vi "室外Otsu.vi"(11 "火焰占比系数":dbl(slide)=0.9 min=0.0 max=1.0 step=0.01 scale=0.0..1.0 scale format="%1.2f") -> ()   [LabVIEW 2018]
doc: "This example shows how to open, read, and display an AVI file in NI Vision. The VI reads the frames per second property and plays the images back at the rate specified by the AVI file."
uses:
  <vilib>/vision/NI_Vision_Development_Module.lvlib
  Dll/fire_Otsu.dll
panel:
  in  "保存":bool
  out "像素当量单位":string
  out "像素当量":string
  in  "清除叠加火焰":bool
  out "总像素":dbl
  out "叠加像素源":u8[][](array[numeric])
  in  "暂停按钮":bool
  out "帧数据":T1
  out "导入像素当量":bool
  in  "火焰详细参数":bool
  out "叠加实际字符串":string
  out "单帧实际字符串":string
  out "叠加像素字符串":string
  out "单帧像素字符串":string
  out "火焰帧数":string
  out "叠加部分":string
  out "单帧部分":string
  in  "单帧回看":bool
  in  "返回":bool
  out "火焰分割":T2(plugin-control)
  out "单幅画面":T2(plugin-control) caption="单帧画面"
  in  "帧数计数":i32(slide) max=241 scale=-1.1..241.0
  in  "程序停止":bool
  out "原图":T2(plugin-control)
  out "火焰叠加":T2(plugin-control)
  # "基于Otsu的最大类间方法火焰分割"
  # "火焰参数"
  # "参\n数\n设\n置"
  # "说明：\n火焰实际面积的单位为标定时的设定的单位，若未进行标注，则不显示实际尺寸。"
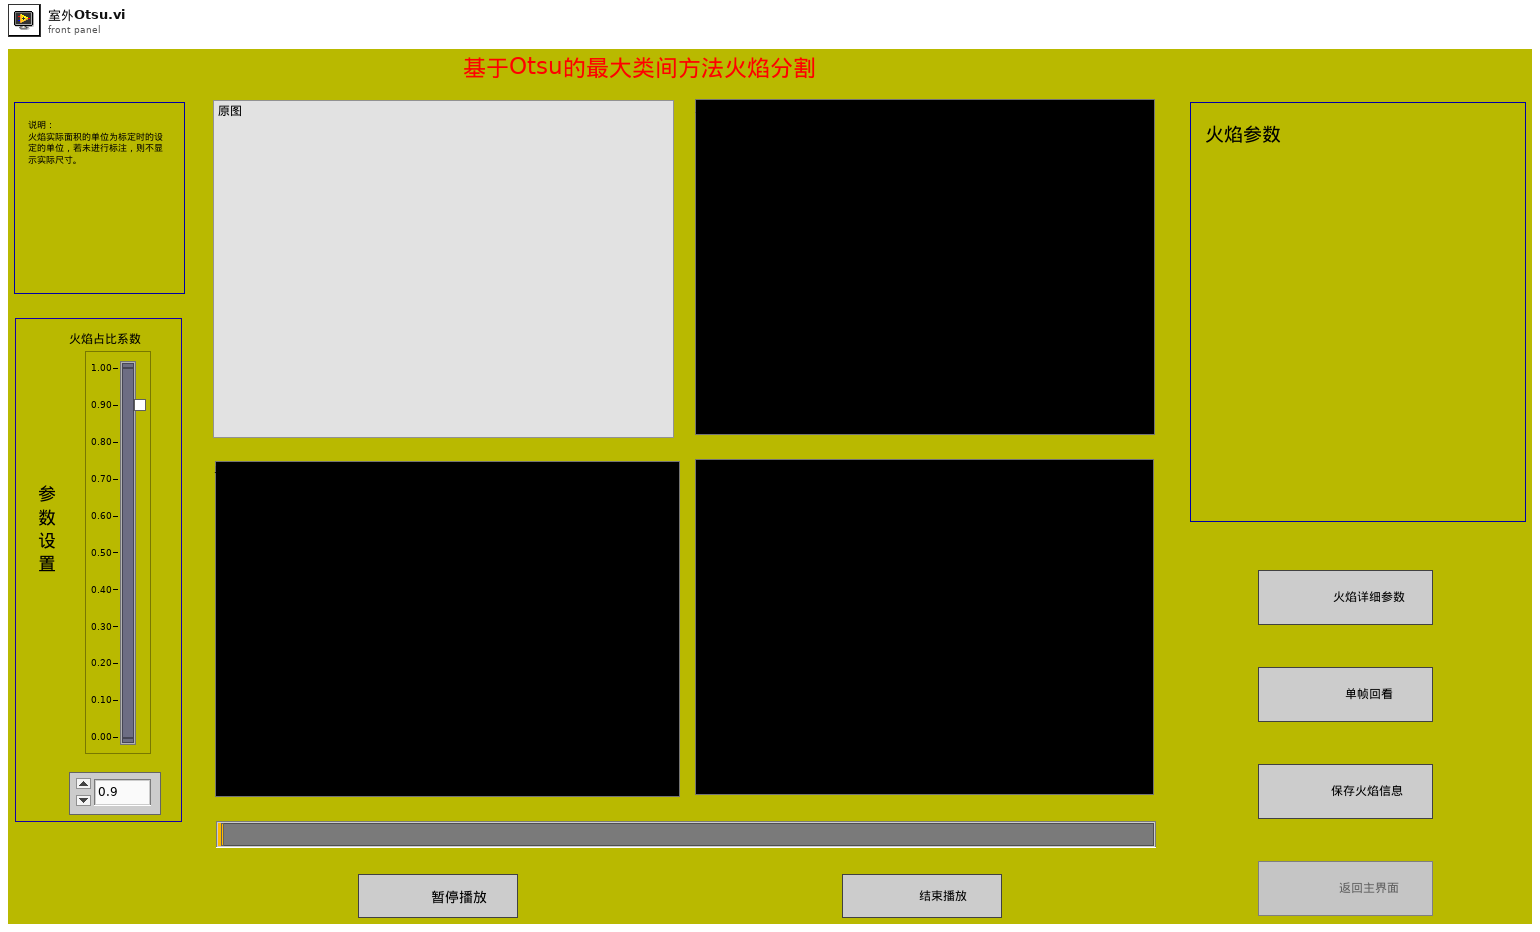
[diagram p1: front panel]
types:
  T1 = cluster{"Width":u32, "Height":u32, "Frames Per Second":u32, "Codec":string, "Has Data":bool}
  T2 = typedef "IMAQ Image.ctl" = refnum<image>
  T3 = enum8{"Enabled", "Disabled", "Disabled and Grayed Out"}
  T4 = typedef "Image Type" = u32
  T5 = enum32{"Invalid", "Standard", "Closed", "Hidden", "Minimized", "Maximized"}
  T6 = typedef "IMAQ AVI2 Refnum.ctl" = refnum<k20>
  T7 = cluster{"X Size":i32, "Y Size":i32, "% Tolerance":i32}
  T8 = typedef "ROI Descriptor" = cluster{"Global Rectangle":i32[], "Contours":cluster{"ID":enum32{"External", "Internal"}, "Type":u32, "Coordinates":i32[]}[]}
  T9 = cluster{"Area":dbl, "Number of Holes":dbl, "Bounding Rect":cluster{"Left":dbl, "Top":dbl, "Right":dbl, "Bottom":dbl}, "Center of Mass":cluster{"X":dbl, "Y":dbl}, "Orientation":dbl, "Dimensions":cluster{"Width":dbl, "Height":dbl}}[]
  T10 = cluster{"Particle Reports (Pixels)[0]":cluster{"Area":dbl, "Number of Holes":dbl, "Bounding Rect":cluster{"Left":dbl, "Top":dbl, "Right":dbl, "Bottom":dbl}, "Center of Mass":cluster{"X":dbl, "Y":dbl}, "Orientation":dbl, "Dimensions":cluster{"Width":dbl, "Height":dbl}}, "Particle Reports (Pixels)[1]":cluster{"Area":dbl, "Number of Holes":dbl, "Bounding Rect":cluster{"Left":dbl, "Top":dbl, "Right":dbl, "Bottom":dbl}, "Center of Mass":cluster{"X":dbl, "Y":dbl}, "Orientation":dbl, "Dimensions":cluster{"Width":dbl, "Height":dbl}}, "Particle Reports (Pixels)[2]":cluster{"Area":dbl, "Number of Holes":dbl, "Bounding Rect":cluster{"Left":dbl, "Top":dbl, "Right":dbl, "Bottom":dbl}, "Center of Mass":cluster{"X":dbl, "Y":dbl}, "Orientation":dbl, "Dimensions":cluster{"Width":dbl, "Height":dbl}}, "Particle Reports (Pixels)[3]":cluster{"Area":dbl, "Number of Holes":dbl, "Bounding Rect":cluster{"Left":dbl, "Top":dbl, "Right":dbl, "Bottom":dbl}, "Center of Mass":cluster{"X":dbl, "Y":dbl}, "Orientation":dbl, "Dimensions":cluster{"Width":dbl, "Height":dbl}}, "Particle Reports (Pixels)[4]":cluster{"Area":dbl, "Number of Holes":dbl, "Bounding Rect":cluster{"Left":dbl, "Top":dbl, "Right":dbl, "Bottom":dbl}, "Center of Mass":cluster{"X":dbl, "Y":dbl}, "Orientation":dbl, "Dimensions":cluster{"Width":dbl, "Height":dbl}}, "Particle Reports (Pixels)[5]":cluster{"Area":dbl, "Number of Holes":dbl, "Bounding Rect":cluster{"Left":dbl, "Top":dbl, "Right":dbl, "Bottom":dbl}, "Center of Mass":cluster{"X":dbl, "Y":dbl}, "Orientation":dbl, "Dimensions":cluster{"Width":dbl, "Height":dbl}}, "Particle Reports (Pixels)[6]":cluster{"Area":dbl, "Number of Holes":dbl, "Bounding Rect":cluster{"Left":dbl, "Top":dbl, "Right":dbl, "Bottom":dbl}, "Center of Mass":cluster{"X":dbl, "Y":dbl}, "Orientation":dbl, "Dimensions":cluster{"Width":dbl, "Height":dbl}}, "Particle Reports (Pixels)[7]":cluster{"Area":dbl, "Number of Holes":dbl, "Bounding Rect":cluster{"Left":dbl, "Top":dbl, "Right":dbl, "Bottom":dbl}, "Center of Mass":cluster{"X":dbl, "Y":dbl}, "Orientation":dbl, "Dimensions":cluster{"Width":dbl, "Height":dbl}}, "Particle Reports (Pixels)[8]":cluster{"Area":dbl, "Number of Holes":dbl, "Bounding Rect":cluster{"Left":dbl, "Top":dbl, "Right":dbl, "Bottom":dbl}, "Center of Mass":cluster{"X":dbl, "Y":dbl}, "Orientation":dbl, "Dimensions":cluster{"Width":dbl, "Height":dbl}}}
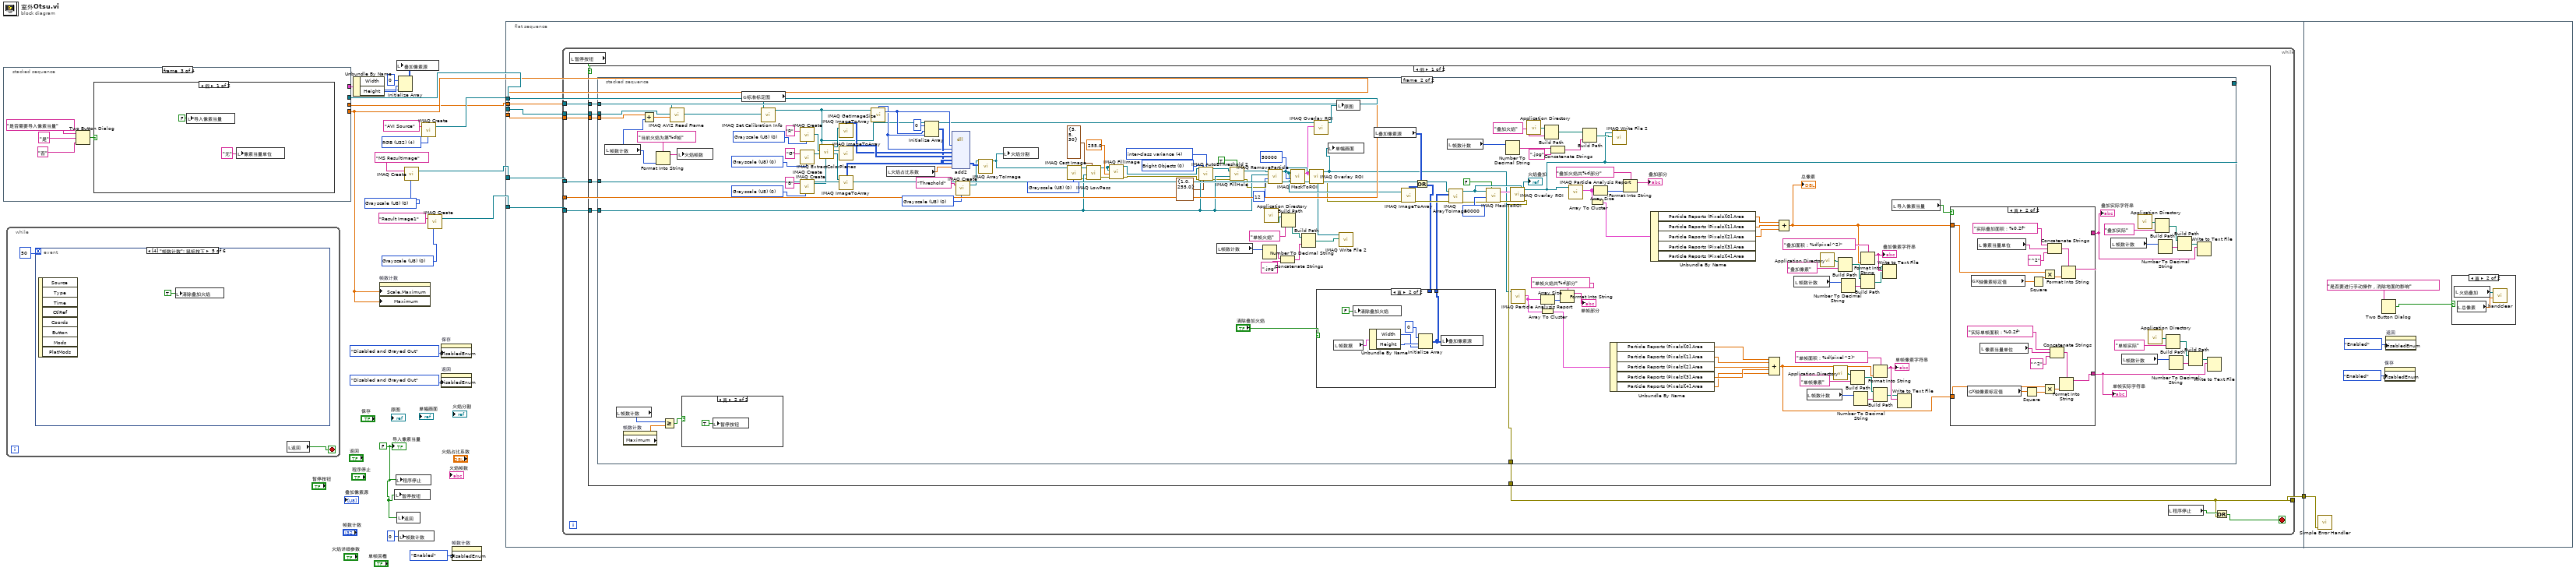
[diagram p0: block diagram]
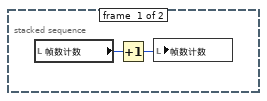
[diagram p2: hidden frame]
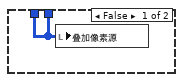
[diagram p3: hidden frame]
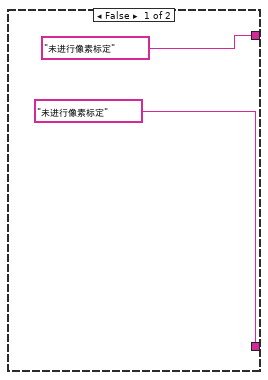
[diagram p5: hidden frame]
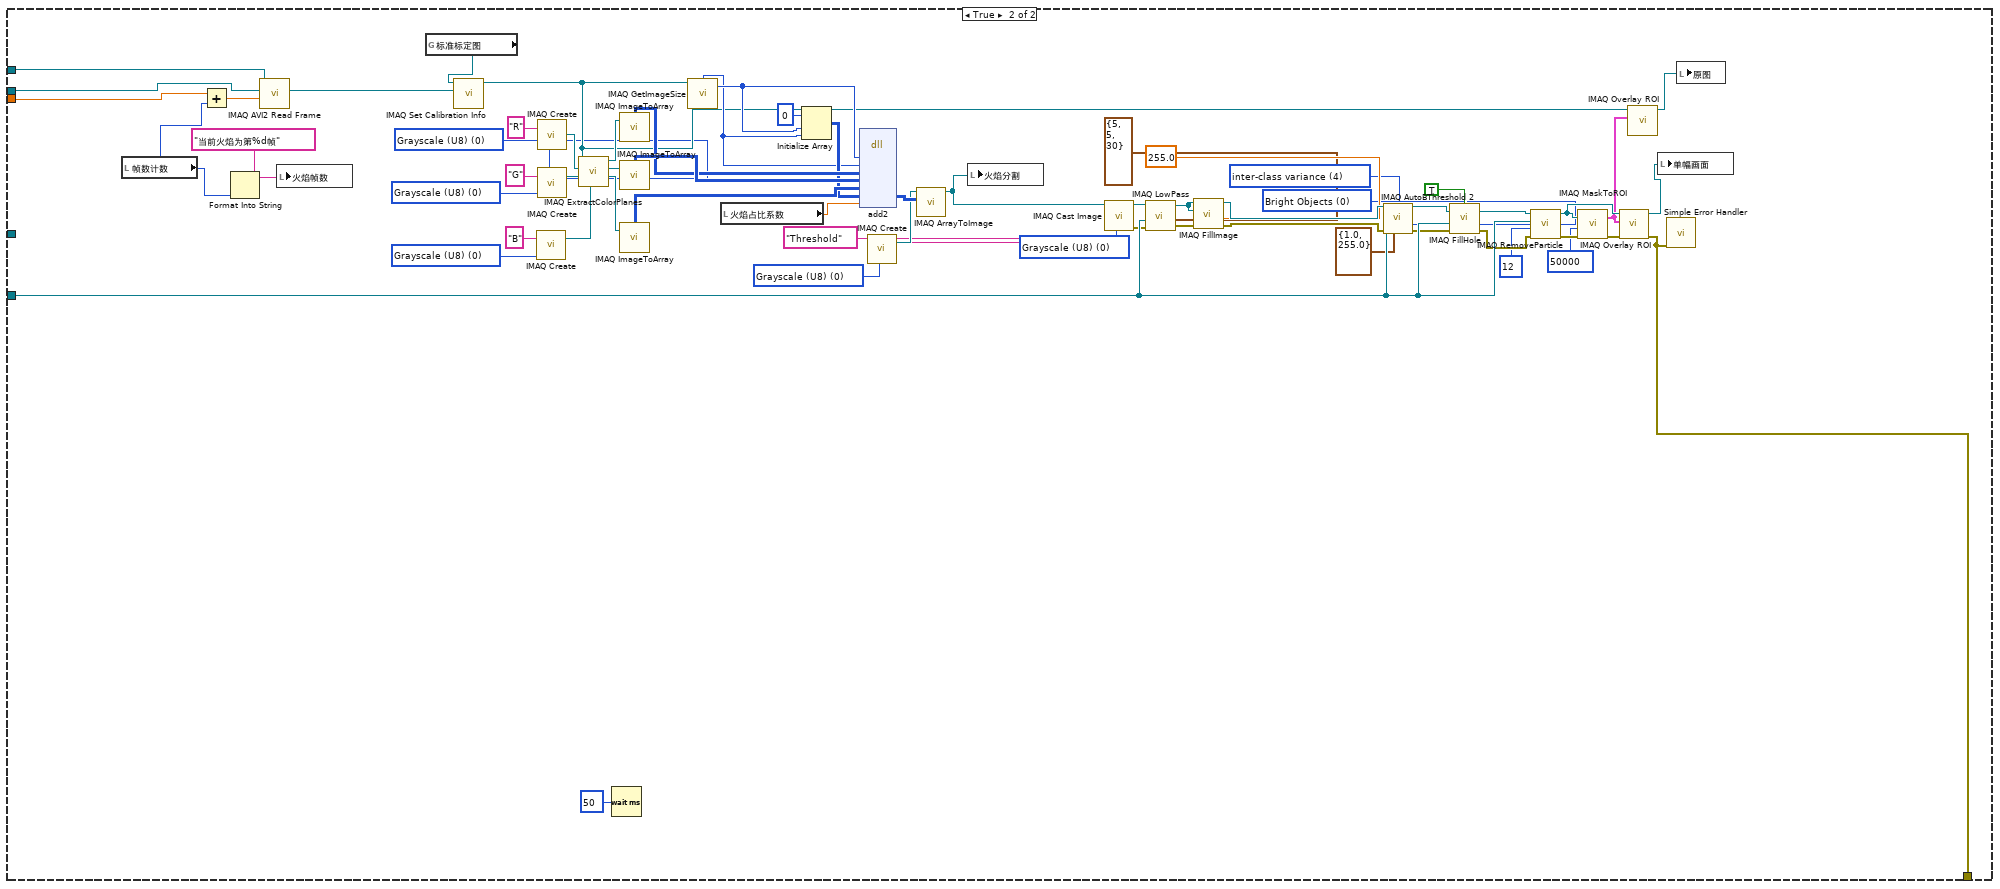
[diagram p6: hidden frame]
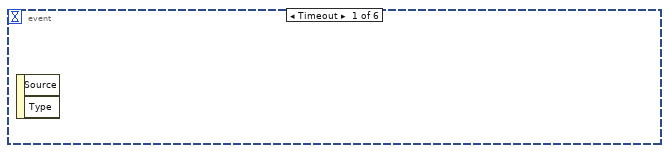
[diagram p8: hidden frame]
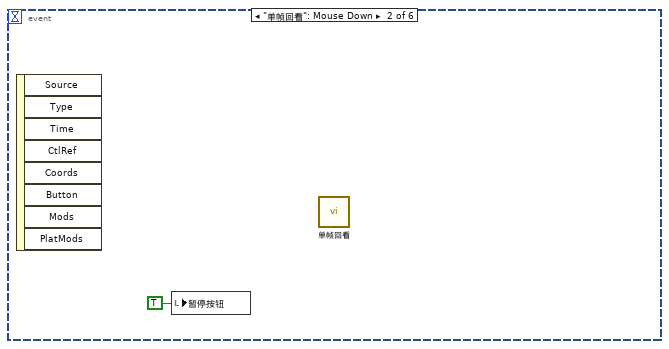
[diagram p9: hidden frame]
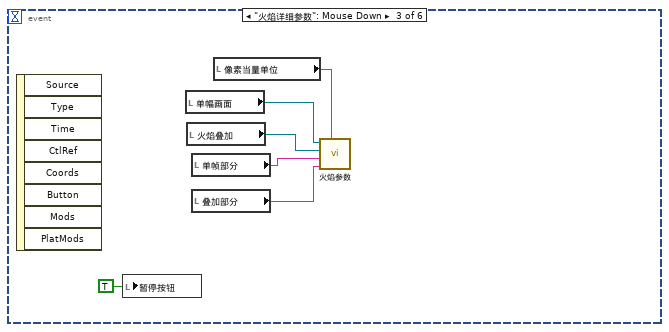
[diagram p10: hidden frame]
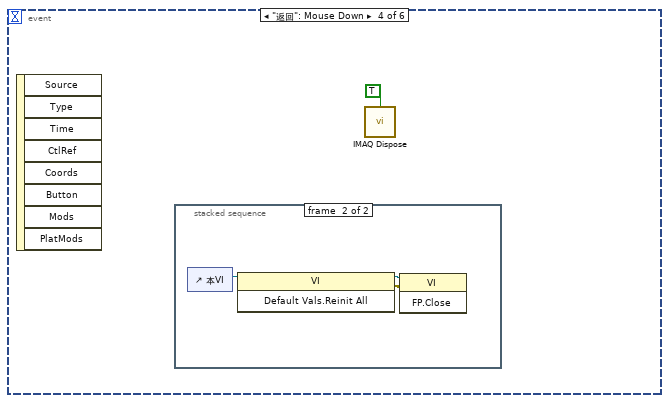
[diagram p11: hidden frame]
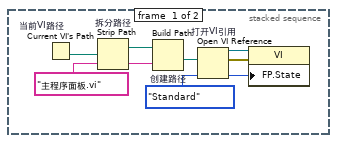
[diagram p12: hidden frame]
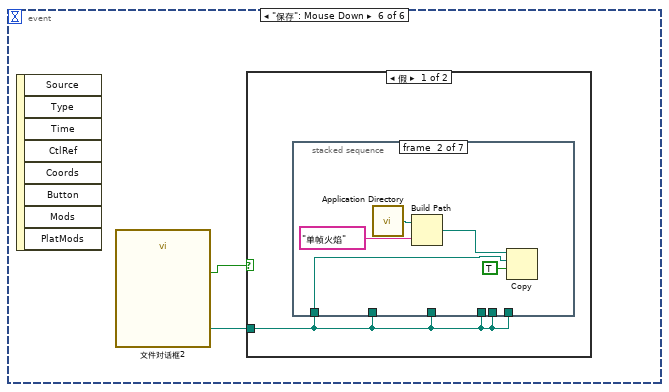
[diagram p13: hidden frame]
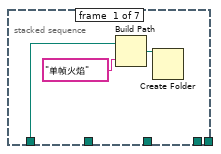
[diagram p14: hidden frame]
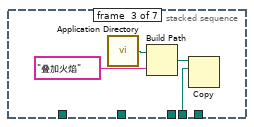
[diagram p15: hidden frame]
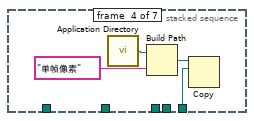
[diagram p16: hidden frame]
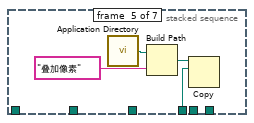
[diagram p17: hidden frame]
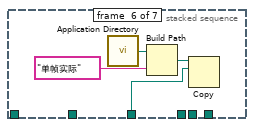
[diagram p18: hidden frame]
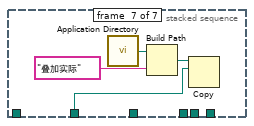
[diagram p19: hidden frame]
diagram:
  w17 = T4 0 items=["Grayscale (U8)", "Grayscale (I16)", "Grayscale (SGL)", "Complex (CSG)", "RGB (U32)", "HSL (U32)", "RGB (U64)", "Grayscale (U16)"] ("Image Type")
  w18 = T4 0 items=["Grayscale (U8)", "Grayscale (I16)", "Grayscale (SGL)", "Complex (CSG)", "RGB (U32)", "HSL (U32)", "RGB (U64)", "Grayscale (U16)"] ("Image Type")
  w20 = T4 4 items=["Grayscale (U8)", "Grayscale (I16)", "Grayscale (SGL)", "Complex (CSG)", "RGB (U32)", "HSL (U32)", "RGB (U64)", "Grayscale (U16)"] ("Image Type")
  w12 = FALSE ("导入像素当量")
  n1 = stacked-sequence {
    tunnel: [_ w31 _ _] -> w6
    tunnel: [_ w30 _ _] -> w5
    tunnel: [_ w29 _ _] -> w4
    tunnel: [_ w28 _ _] -> w22
    frame #0 {
      n2 = One Button Dialog(message="请选择室外火焰视频" ("消息"), button name ("OK")="确定" ("按钮名称（“确定”）")) -> ()  [unwired: 1 out]
    }
    frame #1 {
      n3 = control-ref of="本VI"() -> (w27:refnum<vi>)
      n4 = property class="VI"(reference=w27, "FP.State"=T5."Hidden" ("前面板窗口:状态")) -> ()  [unwired: 1 in, 2 out]
      n5 = call "帧数选择.vi"() -> ("AVI Refnum"=w31:T6, "初始帧"=w29:dbl, "Frame Data"=w28:T1, "结束帧"=w30:dbl)  [unwired: 5 in, 1 out]
      "帧数据" <- w28
    }
    frame #2 {
      n6 = Two Button Dialog(message="是否需要导入像素当量" ("消息"), 1:"否" ("F按钮名称（“取消”）"), 2:"是" ("T按钮名称（“确定”）")) -> (T button?=w32:bool)
      n7 = case shown="假" w32 {
        frame False {
          n8 = local write "导入像素当量"(FALSE ("导入像素当量")) -> ()
          n9 = local write "像素当量单位"("无" ("像素当量单位")) -> ()
        }
        frame True {
          n10 = stacked-sequence {
            frame #0 {
              n11 = call "文件对话框"("default name"="请选择像素当量") -> ("selected path"=w40:path)  [unwired: 11 in, 3 out]
              n12 = Read from Text File(file (use dialog)=w40) -> (text=w41:string)  [unwired: 3 in, 3 out]
              "像素当量" <- w41
              n13 = Fract/Exp String To Number(string=w41) -> (number=w42:dbl)  [unwired: 3 in, 1 out]
              n14 = local write "导入像素当量"(TRUE ("导入像素当量")) -> ()
              n15 = global write "全局变量.vi" "X轴像素标定值"(w42) -> ()
              n16 = global write "全局变量.vi" "Y轴像素标定值"(w42) -> ()
            }
            frame #1 {
              n17 = invoke on="像素当量" class="Str" method="Get Nth Line"("index"=u32 2 ("行索引")) -> (error out=w43:errorcluster, "text"=w44:string)  [unwired: 6 in, 5 out]
              n18 = case shown="错误" w43 {
                selector: w43 -> [_ w49]
                tunnel: w44 -> [w46 _]
                frame No Error {
                  "像素当量单位" <- w46
                }
                frame Error {
                  n19 = call <vilib>:"Simple Error Handler.vi"("error in (no error)"=w49) -> ()  [unwired: 4 in, 5 out]
                  n20 = local write "像素当量单位"("无" ("像素当量单位")) -> ()
                  n21 = One Button Dialog(message="导入像素当量单位时出错，\n请检查导入文件是否正确。" ("消息")) -> ()  [unwired: 1 in, 1 out]
                }
              }
            }
          }
        }
      }
    }
    frame #3 {
      n22 = flat-sequence {
        frame #0 {
          n23 = control-ref of="本VI"() -> (w51:refnum<vi>)
          n24 = property class="VI"(reference=w51, "FP.State"=T5."Standard" ("前面板窗口:状态")) -> ()  [unwired: 1 in, 2 out]
        }
        frame #1 {
          n25 = Wait (ms)(milliseconds to wait=u32 200 ("等待时间（毫秒）")) -> ()  [unwired: 1 out]
        }
      }
    }
  }
  n26 = while {
    stop <- w53 stop-if-true
    n27 = event "事件结构" shown="[4] \"帧数计数\": 鼠标按下" {
      selector: _ -> [_ _ _ _ _ _]
      dyn-events: _ -> [_ _ _ _ _ _]
      timeout: 50 -> [_ _ _ _ _ _]
      event Timeout {
        n28 = event-data() -> ()  [unwired: 1 in, 2 out]
      }
      event "单帧回看": Mouse Down {
        n29 = event-data() -> ()  [unwired: 1 in, 8 out]
        n30 = local write "暂停按钮"(TRUE ("暂停按钮")) -> ()
        n31 = call "单帧回看.vi"() -> ()  [unwired: 28 in]
      }
      event "火焰详细参数": Mouse Down {
        n32 = event-data() -> ()  [unwired: 1 in, 8 out]
        n33 = local write "暂停按钮"(TRUE ("暂停按钮")) -> ()
        n34 = local read "单幅画面"() -> (w59:T2)
        n35 = local read "火焰叠加"() -> (w58:T2)
        n36 = local read "单帧部分"() -> (w61:string)
        n37 = local read "叠加部分"() -> (w60:string)
        n38 = local read "像素当量单位"() -> (w56:string)
        n39 = call "火焰参数.vi"("像素当量单位"=w56, 8:w60, 9:w61, "Image 2"=w58, "Image"=w59) -> ()  [unwired: 7 in]
      }
      event "返回": Mouse Down {
        n40 = event-data() -> ()  [unwired: 1 in, 8 out]
        n41 = stacked-sequence {
          frame #0 {
            n42 = Current VI's Path "当前VI路径"() -> (path=w67:path)
            n43 = Strip Path "拆分路径"(path=w67) -> (stripped path=w69:path)  [unwired: 1 out]
            n44 = Build Path "创建路径"(base path=w69, name or relative path="主程序面板.vi" ("名称或相对路径")) -> (appended path=w68:path)
            n45 = Open VI Reference "打开VI引用"(vi path=w68) -> (vi reference=w66:refnum<vi>, error out=w65:errorcluster)  [unwired: 5 in]
            n46 = property class="VI"(reference=w66, error in=w65, "FP.State"=T5."Standard" ("前面板窗口:状态")) -> ()  [unwired: 2 out]
          }
          frame #1 {
            n47 = control-ref of="本VI"() -> (w70:refnum<vi>)
            n48 = invoke class="VI" method="Default Vals.Reinit All"(reference=w70) -> (reference out=w71:refnum<vi>, error out=w72:errorcluster)  [unwired: 2 in, 1 out]
            n49 = invoke class="VI" method="FP.Close"(reference=w71, error in=w72) -> ()  [unwired: 1 in, 3 out]
          }
        }
        n50 = call "IMAQ Dispose"("All Images? (No)"=TRUE) -> ()  [unwired: 2 in, 4 out]
      }
      event "帧数计数": Mouse Down {
        n51 = event-data() -> ()  [unwired: 1 in, 8 out]
        n52 = local write "清除叠加火焰"(TRUE ("清除叠加火焰")) -> ()
      }
      event "保存": Mouse Down {
        n53 = event-data() -> ()  [unwired: 1 in, 8 out]
        n54 = call "文件对话框2"() -> ("selected path"=w74:path, "cancelled"=w75:bool)  [unwired: 12 in, 2 out]
        n55 = case shown="假" w75 {
          tunnel: w74 -> [w76 _]
          frame False {
            n56 = stacked-sequence {
              tunnel: w76 -> [w77 w81 _ _ _ _ _]
              tunnel: w76 -> [_ _ w86 _ _ _ _]
              tunnel: w76 -> [_ _ _ w90 _ _ _]
              tunnel: w76 -> [_ _ _ _ w94 _ _]
              tunnel: w76 -> [_ _ _ _ _ w98 _]
              tunnel: w76 -> [_ _ _ _ _ _ w101]
              frame #0 {
                n57 = Build Path(base path=w77, name or relative path="单帧火焰" ("名称或相对路径")) -> (appended path=w79:path)
                n58 = Create Folder(path (use dialog)=w79) -> ()  [unwired: 2 in, 3 out]
              }
              frame #1 {
                n59 = call <vilib>:"Application Directory.vi"() -> ("Application Directory"=w84:path)
                n60 = Build Path(base path=w84, name or relative path="单帧火焰" ("名称或相对路径")) -> (appended path=w82:path)
                n61 = Copy(9:TRUE ("覆盖(F)"), 10:w81, 11:w82) -> ()  [unwired: 2 in, 3 out]
              }
              frame #2 {
                n62 = call <vilib>:"Application Directory.vi"() -> ("Application Directory"=w87:path)
                n63 = Build Path(base path=w87, name or relative path="叠加火焰" ("名称或相对路径")) -> (appended path=w88:path)
                n64 = Copy(10:w86, 11:w88) -> ()  [unwired: 3 in, 3 out]
              }
              frame #3 {
                n65 = call <vilib>:"Application Directory.vi"() -> ("Application Directory"=w91:path)
                n66 = Build Path(base path=w91, name or relative path="单帧像素" ("名称或相对路径")) -> (appended path=w92:path)
                n67 = Copy(10:w90, 11:w92) -> ()  [unwired: 3 in, 3 out]
              }
              frame #4 {
                n68 = call <vilib>:"Application Directory.vi"() -> ("Application Directory"=w95:path)
                n69 = Build Path(base path=w95, name or relative path="叠加像素" ("名称或相对路径")) -> (appended path=w96:path)
                n70 = Copy(10:w94, 11:w96) -> ()  [unwired: 3 in, 3 out]
              }
              frame #5 {
                n71 = call <vilib>:"Application Directory.vi"() -> ("Application Directory"=w99:path)
                n72 = Build Path(base path=w99, name or relative path="单帧实际" ("名称或相对路径")) -> (appended path=w100:path)
                n73 = Copy(10:w98, 11:w100) -> ()  [unwired: 3 in, 3 out]
              }
              frame #6 {
                n74 = call <vilib>:"Application Directory.vi"() -> ("Application Directory"=w103:path)
                n75 = Build Path(base path=w103, name or relative path="叠加实际" ("名称或相对路径")) -> (appended path=w104:path)
                n76 = Copy(10:w101, 11:w104) -> ()  [unwired: 3 in, 3 out]
              }
            }
          }
          frame True {
          }
        }
      }
    }
    n77 = local read "返回"() -> (w53:bool)
  }
  n78 = Unbundle By Name(w22) -> ("Width"=w14:u32, "Height"=w15:u32)
  n79 = property on="帧数计数" class="Slide (严格)"("Scale.Maximum"=w5, "Maximum"=w5) -> ()  [unwired: 2 in, 2 out]
  n80 = local write "暂停按钮"(w12) -> ()
  n81 = local write "程序停止"(w12) -> ()
  n82 = local write "返回"(w12) -> ()
  n83 = Initialize Array(u8 0 ("元素"), w15, w14) -> (w10:u8[][])
  n84 = local write "叠加像素源"(w10) -> ()
  n85 = local write "帧数计数"(0 ("帧数计数")) -> ()
  n86 = call "IMAQ Create"("Image Name"="MS ResultImage", "Image Type"=w17) -> ("New Image"=w7:T2)  [unwired: 2 in, 2 out]
  n87 = call "IMAQ Create"("Image Name"="AVI Source", "Image Type"=w20) -> ("New Image"=w9:T2)  [unwired: 2 in, 2 out]
  n88 = call "IMAQ Create"("Image Name"="Result Image1", "Image Type"=w18) -> ("New Image"=w8:T2)  [unwired: 2 in, 2 out]
  n89 = property on="保存" class="Bool (严格)"("DisabledEnum"=T3."Disabled and Grayed Out" ("禁用")) -> ()  [unwired: 2 in, 2 out]
  n90 = property on="返回" class="Bool (严格)"("DisabledEnum"=T3."Disabled and Grayed Out" ("禁用")) -> ()  [unwired: 2 in, 2 out]
  n91 = property on="帧数计数" class="Slide (严格)"("DisabledEnum"=T3."Enabled" ("禁用")) -> ()  [unwired: 2 in, 2 out]
  n92 = flat-sequence {
    tunnel: w9 -> [w111]
    tunnel: w8 -> [w110]
    tunnel: w7 -> [w109]
    tunnel: w6 -> [w108]
    tunnel: w5 -> [w107]
    tunnel: w4 -> [w106]
    tunnel: [w105] -> w3
    tunnel: w3 -> [w368]
    frame #0 {
      n93 = while {
        tunnel: w111 -> [w118]
        tunnel: w110 -> [w117]
        tunnel: w109 -> [w116]
        tunnel: w108 -> [w115]
        tunnel: w107 -> [_]
        tunnel: w106 -> [w120]
        tunnel: [w112] -> w105
        stop <- w113 stop-if-true
        n94 = local read "暂停按钮"() -> (w119:bool)
        n95 = case shown="假" w119 {
          tunnel: w116 -> [w126 _]
          tunnel: w117 -> [w125 w362]
          tunnel: w118 -> [w124 w364]
          tunnel: w115 -> [w123 w365]
          tunnel: w120 -> [w122 w363]
          tunnel: [w121 w304] -> w112
          frame False {
            n96 = stacked-sequence {
              tunnel: w126 -> [_ w275]
              tunnel: w125 -> [_ w274]
              tunnel: w124 -> [_ w273]
              tunnel: w123 -> [_ w149]
              tunnel: w122 -> [_ w148]
              tunnel: [_ w141] -> w121
              tunnel: [_ w137] -> _
              frame #0 {
                n97 = local read "帧数计数"() -> (w128:i32)
                n98 = Increment(x=w128) -> (x+1=w127:i32)
                n99 = local write "帧数计数"(w127) -> ()
              }
              frame #1 {
                w224 = T4 0 items=["Grayscale (U8)", "Grayscale (I16)", "Grayscale (SGL)", "Complex (CSG)", "RGB (U32)", "HSL (U32)", "RGB (U64)", "Grayscale (U16)"] ("Image Type")
                w231 = T4 0 items=["Grayscale (U8)", "Grayscale (I16)", "Grayscale (SGL)", "Complex (CSG)", "RGB (U32)", "HSL (U32)", "RGB (U64)", "Grayscale (U16)"] ("Image Type")
                w232 = T4 0 items=["Grayscale (U8)", "Grayscale (I16)", "Grayscale (SGL)", "Complex (CSG)", "RGB (U32)", "HSL (U32)", "RGB (U64)", "Grayscale (U16)"] ("Image Type")
                w233 = T4 0 items=["Grayscale (U8)", "Grayscale (I16)", "Grayscale (SGL)", "Complex (CSG)", "RGB (U32)", "HSL (U32)", "RGB (U64)", "Grayscale (U16)"] ("Image Type")
                w265 = u32 0 items=["Bright Objects", "Dark Objects"] ("Look For (Bright Objects)")
                w268 = 4 items=["clustering", "entropy", "metric", "moments", "inter-class variance"] ("Method")
                w269 = T4 0 items=["Grayscale (U8)", "Grayscale (I16)", "Grayscale (SGL)", "Complex (CSG)", "RGB (U32)", "HSL (U32)", "RGB (U64)", "Grayscale (U16)"] ("Image Type")
                n100 = local read "帧数计数"() -> (w147:i32)
                n101 = local read "帧数计数"() -> (w145:i32)
                n102 = property on="帧数计数" class="Slide (严格)"() -> ("Maximum"=w144:dbl)  [unwired: 2 in, 2 out]
                n103 = Add(x=w148, y=w147) -> (x+y=w219:dbl)
                n104 = Format Into String(format string="当前火焰为第%d帧" ("初始字符串"), w147) -> (resulting string=w136:string)  [unwired: 2 in, 1 out]
                n105 = Greater Or Equal?(x=w145, y=w144) -> (x >= y?=w143:bool)
                n106 = call "IMAQ AVI2 Read Frame"("Frame Number"=w219, "Image"=w273, "AVI Refnum"=w149) -> ("Image Out"=w197:T2)  [unwired: 1 in, 7 out]
                n107 = local write "火焰帧数"(w136) -> ()
                n108 = case shown="真" w143 {
                  frame False {
                  }
                  frame True {
                    n109 = local write "暂停按钮"(TRUE ("暂停按钮")) -> ()
                  }
                }
                n110 = global read "全局变量.vi" "标准标定图"() -> (w196:T2)
                n111 = call "IMAQ Set Calibration Info"("Image Dst"=w197, "Image Src"=w196) -> ("Calibrated Image"=w198:T2)  [unwired: 8 in, 1 out]
                n112 = call "IMAQ Create"("Image Name"="B", "Image Type"=w231) -> ("New Image"=w242:T2)  [unwired: 3 in, 1 out]
                n113 = call "IMAQ Create"("Image Name"="R", "Image Type"=w233) -> ("New Image"=w240:T2)  [unwired: 3 in, 1 out]
                n114 = call "IMAQ Create"("Image Name"="G", "Image Type"=w232) -> ("New Image"=w238:T2)  [unwired: 3 in, 1 out]
                n115 = call "IMAQ ExtractColorPlanes"("Blue or Luma or Val or Inten Plane"=w242, "Green or Sat Plane"=w238, "Red or Hue Plane"=w240, "Image Src"=w198) -> ("Blue or Luma or Val or Inten Plane out"=w234:T2, "Green or Sat Plane out"=w235:T2, "Red or Hue Plane out"=w236:T2)  [unwired: 4 in, 1 out]
                n116 = call "IMAQ ImageToArray"("Image"=w236) -> ("Image Pixels (U8)"=w228:u8[][])  [unwired: 3 in, 4 out]
                n117 = call "IMAQ ImageToArray"("Image"=w235) -> ("Image Pixels (U8)"=w230:u8[][])  [unwired: 3 in, 4 out]
                n118 = call "IMAQ ImageToArray"("Image"=w234) -> ("Image Pixels (U8)"=w229:u8[][])  [unwired: 3 in, 4 out]
                n119 = call "IMAQ GetImageSize"("Image"=w198) -> ("Y Resolution"=w221:i32, "X Resolution"=w220:i32)  [unwired: 3 in, 1 out]
                n120 = local read "火焰占比系数"() -> (w135:dbl)
                n121 = Initialize Array ("data")(u8 0, w221, w220) -> (w223:u8[][])
                n122 = dll-call lib="PTH2Aabs DsdhProgramme_GuShiJu火焰分割Dll\nfire_Otsu.dll" fn="add2"("rows"=w221, "cols"=w220, "ImageR"=w228, "ImageG"=w230, "ImageB"=w229, "data"=w223, "a"=w135) -> ("data"=w227:u8[][])  [unwired: 10 in, 2 out]
                n123 = call "IMAQ Create"("Image Name"="Threshold", "Image Type"=w224) -> ("New Image"=w226:T2)  [unwired: 3 in, 1 out]
                n124 = call "IMAQ ArrayToImage"("Image Pixels (U8)"=w227, "Image"=w226) -> ("Image Out"=w134:T2)  [unwired: 8 in, 1 out]
                n125 = local write "火焰分割"(w134) -> ()
                n126 = call "IMAQ Cast Image"("Image Type"=w269, "Image Src"=w134) -> ("error out"=w248:errorcluster, "Image Dst Out"=w244:T2)  [unwired: 8 in]
                n127 = call "IMAQ LowPass"("Image Src"=w244, "Size & Tolerance"=T7 {"X Size"=5, "Y Size"=5, "% Tolerance"=30}, "Image Dst"=w274, "error in (no error)"=w248) -> ("Image Dst Out"=w252:T2, "error out"=w256:errorcluster)  [unwired: 3 in]
                n128 = call "IMAQ FillImage"("error in (no error)"=w256, "Pixel Value (U8, U16, I16, Float)"=sgl 255.0, "Image Mask"=w252, "Image"=w252) -> ("error out"=w255:errorcluster, "Image Out"=w251:T2)  [unwired: 6 in]
                n129 = call "IMAQ AutoBThreshold 2"("Image Src"=w251, "Look For (Bright Objects)"=w265, "Method (clustering)"=w268, "Image Dst"=w274, "error in (no error)"=w255, "Threshold Limits"=cluster{"Lower value":sgl, "Upper value":sgl} {"Lower value"=1.0, "Upper value"=255.0}) -> ("Image Dst Out"=w254:T2, "error out"=w267:errorcluster)  [unwired: 2 in, 6 out]
                n130 = local read "帧数计数"() -> (w187:i32)
                n131 = call "IMAQ FillHole"("error in (no error)"=w267, "Image Dst"=w274, "Image Src"=w254, "Connectivity 4/8 (8)"=TRUE) -> ("error out"=w263:errorcluster, "Image Dst Out"=w253:T2)  [unwired: 2 in]
                n132 = Number To Decimal String(number=w187) -> (decimal integer string=w182:string)  [unwired: 1 in]
                n133 = call <vilib>:"Application Directory.vi"() -> ("Application Directory"=w195:path)
                n134 = call "IMAQ RemoveParticle"("error in (no error)"=w263, "Number of Erosion"=12, "Image Dst"=w274, "Image Src"=w253) -> ("error out"=w261:errorcluster, "Image Dst Out"=w250:T2)  [unwired: 6 in]
                n135 = Concatenate Strings(w182, ".jpg" ("字符串")) -> (w181:string)
                n136 = Build Path(base path=w195, name or relative path="单帧火焰" ("名称或相对路径")) -> (appended path=w194:path)
                n137 = call "IMAQ MaskToROI"("Image"=w250, "Max number of vectors in ROI"=50000, "error in (no error)"=w261) -> ("ROI Descriptor"=w200:T8, "error out"=w260:errorcluster)  [unwired: 4 in, 1 out]
                n138 = Build Path(base path=w194, name or relative path=w181) -> (appended path=w193:path)
                n139 = call "IMAQ Overlay ROI"("error in (no error)"=w260, "ROI Descriptor"=w200, "Image"=w250) -> ("error out"=w146:errorcluster, "Image Out"=w132:T2)  [unwired: 7 in]
                n140 = call "IMAQ Overlay ROI"("ROI Descriptor"=w200, "Image"=w198) -> ("Image Out"=w133:T2)  [unwired: 8 in, 1 out]
                n141 = local write "单幅画面"(w132) -> ()
                n142 = local write "原图"(w133) -> ()
                n143 = call-poly "IMAQ Write File 2"("File Path"=w193, "Image"=w132) -> ()  [unwired: 8 in, 2 out]
                n144 = local read "叠加像素源"() -> (w142:u8[][])
                n145 = call "IMAQ ImageToArray"("error in (no error)"=w146, "Image"=w250) -> ("error out"=w247:errorcluster, "Image Pixels (U8)"=w249:u8[][])  [unwired: 2 in, 3 out]
                n146 = Or(x=w142, y=w249) -> (x .or. y?=w131:u8[][])
                n147 = case shown="真" "清除叠加火焰" {
                  tunnel: w131 -> [w276 _]
                  tunnel: [w276 w278] -> w129
                  frame False {
                    n148 = local write "叠加像素源"(w276) -> ()
                  }
                  frame True {
                    n149 = local read "帧数据"() -> (w280:T1)
                    n150 = local write "清除叠加火焰"(FALSE ("清除叠加火焰")) -> ()
                    n151 = Unbundle By Name(w280) -> ("Width"=w281:u32, "Height"=w282:u32)
                    n152 = Initialize Array(0, w282, w281) -> (w278:i32[][])
                    n153 = local write "叠加像素源"(w278) -> ()
                  }
                }
                n154 = local read "帧数计数"() -> (w186:i32)
                n155 = call "IMAQ ArrayToImage"("error in (no error)"=w247, "Image Pixels (U8)"=w129, "Image"=w275) -> ("error out"=w246:errorcluster, "Image Out"=w245:T2)  [unwired: 7 in]
                n156 = call "IMAQ MaskToROI"("External edges only (T)"=FALSE, "Image"=w245, "Max number of vectors in ROI"=50000, "error in (no error)"=w246) -> ("ROI Descriptor"=w272:T8, "error out"=w271:errorcluster)  [unwired: 3 in, 1 out]
                n157 = Number To Decimal String(number=w186) -> (decimal integer string=w185:string)  [unwired: 1 in]
                n158 = call "IMAQ Overlay ROI"("error in (no error)"=w271, "ROI Descriptor"=w272, "Image"=w245) -> ("error out"=w141:errorcluster, "Image Out"=w137:T2)  [unwired: 7 in]
                "火焰叠加" <- w137
                n159 = call "IMAQ Particle Analysis Report"("Image"=w132) -> ("Particle Reports (Pixels)"=w205:T9)  [unwired: 5 in, 5 out]
                n160 = call <vilib>:"Application Directory.vi"() -> ("Application Directory"=w191:path)
                n161 = Array To Cluster(array=w205) -> (cluster=w218:T10)
                n162 = Array Size(array=w205) -> (size(s)=w208:i32)
                n163 = Build Path(base path=w191, name or relative path="叠加火焰" ("名称或相对路径")) -> (appended path=w189:path)
                n164 = Concatenate Strings(w185, ".jpg" ("字符串")) -> (w184:string)
                n165 = Format Into String(format string="单帧火焰共%d部分" ("初始字符串"), w208) -> (resulting string=→"单帧部分":string)  [unwired: 2 in, 1 out]
                n166 = call "IMAQ Particle Analysis Report"("Image"=w137) -> ("Particle Reports (Pixels)"=w201:T9)  [unwired: 5 in, 5 out]
                n167 = Build Path(base path=w189, name or relative path=w184) -> (appended path=w188:path)
                n168 = Array To Cluster(array=w201) -> (cluster=w214:T10)
                n169 = Array Size(array=w201) -> (size(s)=w203:i32)
                n170 = Unbundle By Name(w218) -> ("Particle Reports (Pixels)[0].Area"=w217:dbl, "Particle Reports (Pixels)[1].Area"=w216:dbl, "Particle Reports (Pixels)[2].Area"=w215:dbl, "Particle Reports (Pixels)[3].Area"=w213:dbl, "Particle Reports (Pixels)[4].Area"=w212:dbl)
                n171 = call-poly "IMAQ Write File 2"("File Path"=w188, "Image"=w137) -> ()  [unwired: 8 in, 2 out]
                n172 = Format Into String(format string="叠加火焰共%d部分" ("初始字符串"), w203) -> (resulting string=→"叠加部分":string)  [unwired: 2 in, 1 out]
                n173 = Unbundle By Name(w214) -> ("Particle Reports (Pixels)[0].Area"=w211:dbl, "Particle Reports (Pixels)[1].Area"=w210:dbl, "Particle Reports (Pixels)[2].Area"=w209:dbl)  [unwired: 2 out]
                n174 = Compound Arithmetic op=ADD(w217, w216, w215, w213, w212) -> (w140:dbl)
                n175 = Compound Arithmetic op=ADD(w211, w210, w209) -> (w138:dbl)
                "总像素" <- w138
                n176 = local read "帧数计数"() -> (w170:i32)
                n177 = local read "帧数计数"() -> (w174:i32)
                n178 = call <vilib>:"Application Directory.vi"() -> ("Application Directory"=w171:path)
                n179 = call <vilib>:"Application Directory.vi"() -> ("Application Directory"=w173:path)
                n180 = Build Path(base path=w171, name or relative path="叠加像素" ("字符串")) -> (appended path=w164:path)
                n181 = Number To Decimal String(number=w170) -> (decimal integer string=w162:string)  [unwired: 1 in]
                n182 = Build Path(base path=w173, name or relative path="单帧像素" ("字符串")) -> (appended path=w151:path)
                n183 = Number To Decimal String(number=w174) -> (decimal integer string=w150:string)  [unwired: 1 in]
                n184 = Format Into String(format string="叠加面积：%d(pixel^2)" ("格式字符串"), w138) -> (resulting string=w169:string)  [unwired: 2 in, 1 out]
                "叠加像素字符串" <- w169
                n185 = Build Path(base path=w164, name or relative path=w162) -> (appended path=w163:path)
                n186 = Format Into String(format string="单帧面积：%d(pixel^2)" ("格式字符串"), w140) -> (resulting string=w172:string)  [unwired: 2 in, 1 out]
                "单帧像素字符串" <- w172
                n187 = Build Path(base path=w151, name or relative path=w150) -> (appended path=w152:path)
                n188 = Write to Text File(file (use dialog)=w163, text=w169) -> ()  [unwired: 2 in, 3 out]
                n189 = local read "导入像素当量"() -> (w177:bool)
                n190 = Write to Text File(file (use dialog)=w152, text=w172) -> ()  [unwired: 2 in, 3 out]
                n191 = case shown="真" w177 {
                  tunnel: ["未进行像素标定" w303] -> w166
                  tunnel: w138 -> [_ w300]
                  tunnel: w140 -> [_ w295]
                  tunnel: ["未进行像素标定" w294] -> w139
                  frame False {
                  }
                  frame True {
                    n192 = global read "全局变量.vi" "X轴像素标定值"() -> (w297:dbl)
                    n193 = global read "全局变量.vi" "X轴像素标定值"() -> (w301:dbl)
                    n194 = local read "像素当量单位"() -> (w292:string)
                    n195 = local read "像素当量单位"() -> (w289:string)
                    n196 = Square(x=w297) -> (x^2=w296:dbl)
                    n197 = Square(x=w301) -> (x^2=w302:dbl)
                    n198 = Multiply(x=w300, y=w302) -> (x*y=w299:dbl)
                    n199 = Multiply(x=w295, y=w296) -> (x*y=w298:dbl)
                    n200 = Concatenate Strings("实际叠加面积：%0.2f" ("格式字符串"), w292, "^2" ("字符串")) -> (w290:string)
                    n201 = Concatenate Strings("实际单帧面积：%0.2f" ("格式字符串"), w289, "^2" ("字符串")) -> (w286:string)
                    n202 = Format Into String(format string=w286, w298) -> (resulting string=w294:string)  [unwired: 2 in, 1 out]
                    n203 = Format Into String(format string=w290, w299) -> (resulting string=w303:string)  [unwired: 2 in, 1 out]
                  }
                }
                "单帧实际字符串" <- w139
                "叠加实际字符串" <- w166
                n204 = local read "帧数计数"() -> (w168:i32)
                n205 = local read "帧数计数"() -> (w175:i32)
                n206 = call <vilib>:"Application Directory.vi"() -> ("Application Directory"=w167:path)
                n207 = call <vilib>:"Application Directory.vi"() -> ("Application Directory"=w176:path)
                n208 = Build Path(base path=w167, name or relative path="叠加实际" ("字符串")) -> (appended path=w161:path)
                n209 = Number To Decimal String(number=w168) -> (decimal integer string=w159:string)  [unwired: 1 in]
                n210 = Build Path(base path=w176, name or relative path="单帧实际" ("字符串")) -> (appended path=w157:path)
                n211 = Number To Decimal String(number=w175) -> (decimal integer string=w156:string)  [unwired: 1 in]
                n212 = Build Path(base path=w161, name or relative path=w159) -> (appended path=w158:path)
                n213 = Build Path(base path=w157, name or relative path=w156) -> (appended path=w154:path)
                n214 = Write to Text File(file (use dialog)=w158, text=w166) -> ()  [unwired: 2 in, 3 out]
                n215 = Write to Text File(file (use dialog)=w154, text=w139) -> ()  [unwired: 2 in, 3 out]
              }
            }
          }
          frame True {
            w320 = T4 0 items=["Grayscale (U8)", "Grayscale (I16)", "Grayscale (SGL)", "Complex (CSG)", "RGB (U32)", "HSL (U32)", "RGB (U64)", "Grayscale (U16)"] ("Image Type")
            w318 = T4 0 items=["Grayscale (U8)", "Grayscale (I16)", "Grayscale (SGL)", "Complex (CSG)", "RGB (U32)", "HSL (U32)", "RGB (U64)", "Grayscale (U16)"] ("Image Type")
            w314 = T4 0 items=["Grayscale (U8)", "Grayscale (I16)", "Grayscale (SGL)", "Complex (CSG)", "RGB (U32)", "HSL (U32)", "RGB (U64)", "Grayscale (U16)"] ("Image Type")
            w316 = T4 0 items=["Grayscale (U8)", "Grayscale (I16)", "Grayscale (SGL)", "Complex (CSG)", "RGB (U32)", "HSL (U32)", "RGB (U64)", "Grayscale (U16)"] ("Image Type")
            w308 = u32 0 items=["Bright Objects", "Dark Objects"] ("Look For (Bright Objects)")
            w307 = 4 items=["clustering", "entropy", "metric", "moments", "inter-class variance"] ("Method")
            w305 = T4 0 items=["Grayscale (U8)", "Grayscale (I16)", "Grayscale (SGL)", "Complex (CSG)", "RGB (U32)", "HSL (U32)", "RGB (U64)", "Grayscale (U16)"] ("Image Type")
            n216 = local read "帧数计数"() -> (w329:i32)
            n217 = Add(x=w363, y=w329) -> (x+y=w334:dbl)
            n218 = Format Into String(format string="当前火焰为第%d帧" ("初始字符串"), w329) -> (resulting string=w328:string)  [unwired: 2 in, 1 out]
            n219 = call "IMAQ AVI2 Read Frame"("Frame Number"=w334, "Image"=w364, "AVI Refnum"=w365) -> ("Image Out"=w331:T2)  [unwired: 1 in, 7 out]
            n220 = local write "火焰帧数"(w328) -> ()
            n221 = global read "全局变量.vi" "标准标定图"() -> (w330:T2)
            n222 = call "IMAQ Set Calibration Info"("Image Dst"=w331, "Image Src"=w330) -> ("Calibrated Image"=w332:T2)  [unwired: 8 in, 1 out]
            n223 = call "IMAQ Create"("Image Name"="B", "Image Type"=w318) -> ("New Image"=w348:T2)  [unwired: 3 in, 1 out]
            n224 = call "IMAQ Create"("Image Name"="R", "Image Type"=w316) -> ("New Image"=w347:T2)  [unwired: 3 in, 1 out]
            n225 = call "IMAQ Create"("Image Name"="G", "Image Type"=w314) -> ("New Image"=w346:T2)  [unwired: 3 in, 1 out]
            n226 = call "IMAQ ExtractColorPlanes"("Blue or Luma or Val or Inten Plane"=w348, "Green or Sat Plane"=w346, "Red or Hue Plane"=w347, "Image Src"=w332) -> ("Blue or Luma or Val or Inten Plane out"=w343:T2, "Green or Sat Plane out"=w344:T2, "Red or Hue Plane out"=w345:T2)  [unwired: 4 in, 1 out]
            n227 = Wait (ms)(milliseconds to wait=u32 50 ("等待时间（毫秒）")) -> ()  [unwired: 1 out]
            n228 = call "IMAQ ImageToArray"("Image"=w345) -> ("Image Pixels (U8)"=w340:u8[][])  [unwired: 3 in, 4 out]
            n229 = call "IMAQ ImageToArray"("Image"=w344) -> ("Image Pixels (U8)"=w342:u8[][])  [unwired: 3 in, 4 out]
            n230 = call "IMAQ ImageToArray"("Image"=w343) -> ("Image Pixels (U8)"=w341:u8[][])  [unwired: 3 in, 4 out]
            n231 = call "IMAQ GetImageSize"("Image"=w332) -> ("Y Resolution"=w336:i32, "X Resolution"=w335:i32)  [unwired: 3 in, 1 out]
            n232 = local read "火焰占比系数"() -> (w327:dbl)
            n233 = Initialize Array ("data")(u8 0, w336, w335) -> (w337:u8[][])
            n234 = dll-call lib="PTH2Aabs DsdhProgramme_GuShiJu火焰分割Dll\nfire_Otsu.dll" fn="add2"("rows"=w336, "cols"=w335, "ImageR"=w340, "ImageG"=w342, "ImageB"=w341, "data"=w337, "a"=w327) -> ("data"=w339:u8[][])  [unwired: 10 in, 2 out]
            n235 = call "IMAQ Create"("Image Name"="Threshold", "Image Type"=w320) -> ("New Image"=w338:T2)  [unwired: 3 in, 1 out]
            n236 = call "IMAQ ArrayToImage"("Image Pixels (U8)"=w339, "Image"=w338) -> ("Image Out"=w326:T2)  [unwired: 8 in, 1 out]
            n237 = local write "火焰分割"(w326) -> ()
            n238 = call "IMAQ Cast Image"("Image Type"=w305, "Image Src"=w326) -> ("error out"=w350:errorcluster, "Image Dst Out"=w349:T2)  [unwired: 8 in]
            n239 = call "IMAQ LowPass"("Image Src"=w349, "Size & Tolerance"=T7 {"X Size"=5, "Y Size"=5, "% Tolerance"=30}, "Image Dst"=w362, "error in (no error)"=w350) -> ("Image Dst Out"=w353:T2, "error out"=w357:errorcluster)  [unwired: 3 in]
            n240 = call "IMAQ FillImage"("error in (no error)"=w357, "Pixel Value (U8, U16, I16, Float)"=sgl 255.0, "Image Mask"=w353, "Image"=w353) -> ("error out"=w356:errorcluster, "Image Out"=w352:T2)  [unwired: 6 in]
            n241 = call "IMAQ AutoBThreshold 2"("Image Src"=w352, "Look For (Bright Objects)"=w308, "Method (clustering)"=w307, "Image Dst"=w362, "error in (no error)"=w356, "Threshold Limits"=cluster{"Lower value":sgl, "Upper value":sgl} {"Lower value"=1.0, "Upper value"=255.0}) -> ("Image Dst Out"=w355:T2, "error out"=w361:errorcluster)  [unwired: 2 in, 6 out]
            n242 = call "IMAQ FillHole"("error in (no error)"=w361, "Image Dst"=w362, "Image Src"=w355, "Connectivity 4/8 (8)"=TRUE) -> ("error out"=w360:errorcluster, "Image Dst Out"=w354:T2)  [unwired: 2 in]
            n243 = call "IMAQ RemoveParticle"("error in (no error)"=w360, "Number of Erosion"=12, "Image Dst"=w362, "Image Src"=w354) -> ("error out"=w359:errorcluster, "Image Dst Out"=w351:T2)  [unwired: 6 in]
            n244 = call "IMAQ MaskToROI"("Image"=w351, "Max number of vectors in ROI"=50000, "error in (no error)"=w359) -> ("ROI Descriptor"=w333:T8, "error out"=w358:errorcluster)  [unwired: 4 in, 1 out]
            n245 = call "IMAQ Overlay ROI"("error in (no error)"=w358, "ROI Descriptor"=w333, "Image"=w351) -> ("error out"=w304:errorcluster, "Image Out"=w324:T2)  [unwired: 7 in]
            n246 = call "IMAQ Overlay ROI"("ROI Descriptor"=w333, "Image"=w332) -> ("Image Out"=w325:T2)  [unwired: 8 in, 1 out]
            n247 = local write "单幅画面"(w324) -> ()
            n248 = call <vilib>:"Simple Error Handler.vi"("error in (no error)"=w304) -> ()  [unwired: 4 in, 5 out]
            n249 = local write "原图"(w325) -> ()
          }
        }
        n250 = local read "程序停止"() -> (w114:bool)
        n251 = Or(x=w114, y=w112) -> (x .or. y?=w113:bool)
      }
    }
    frame #1 {
      n252 = call <vilib>:"Simple Error Handler.vi"("error in (no error)"=w368) -> ()  [unwired: 1 in, 8 out]
      n253 = Two Button Dialog(message="是否要进行手动操作，消除地面的影响" ("消息")) -> (T button?=w369:bool)  [unwired: 2 in]
      n254 = property on="保存" class="Bool (严格)"("DisabledEnum"=T3."Enabled" ("禁用")) -> ()  [unwired: 2 in, 2 out]
      n255 = property on="返回" class="Bool (严格)"("DisabledEnum"=T3."Enabled" ("禁用")) -> ()  [unwired: 2 in, 2 out]
      n256 = case shown="真" w369 {
        frame False {
        }
        frame True {
          n257 = local read "火焰叠加"() -> (w372:T2)
          n258 = local read "总像素"() -> (w373:dbl)
          n259 = call "handclear.vi"("总像素"=w373, "Image 3"=w372) -> ()  [unwired: 10 in]
        }
      }
    }
  }
  "导入像素当量" <- w12
